vi "SyntaxCheck.vi"(8 "error in":errorcluster, 11 "Logical Parsed Expression":T1) -> (0 "error out":errorcluster, 1 "Error Index":i32, 2 "Funcion Analizada":string, 3 "Logical Parsed Expression Out":T1)   [LabVIEW 2014, in "SeqLoop.lvlib"]
uses:
  TypeDefs/LogicParsedExpression.ctl
  <vilib>/regexp/Match Regular Expression.xnode
  SeqLoop.lvlib
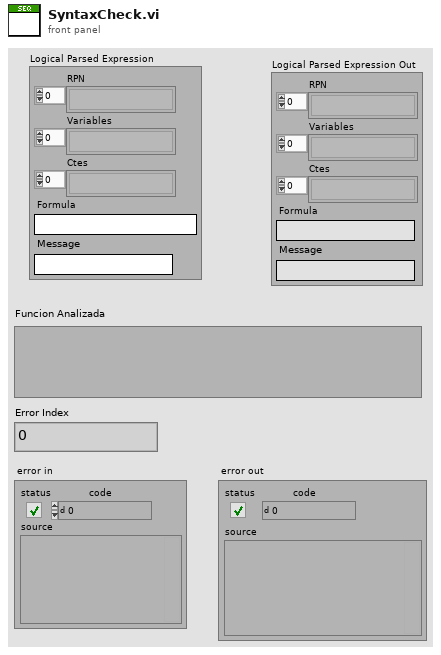
[diagram p1: front panel]
types:
  T1 = typedef "SeqLoop.lvlib/LogicParsedExpression.ctl" = cluster{"RPN ":string[], "Variables":string[], "Ctes":string[], "Formula":string, "Message":string}
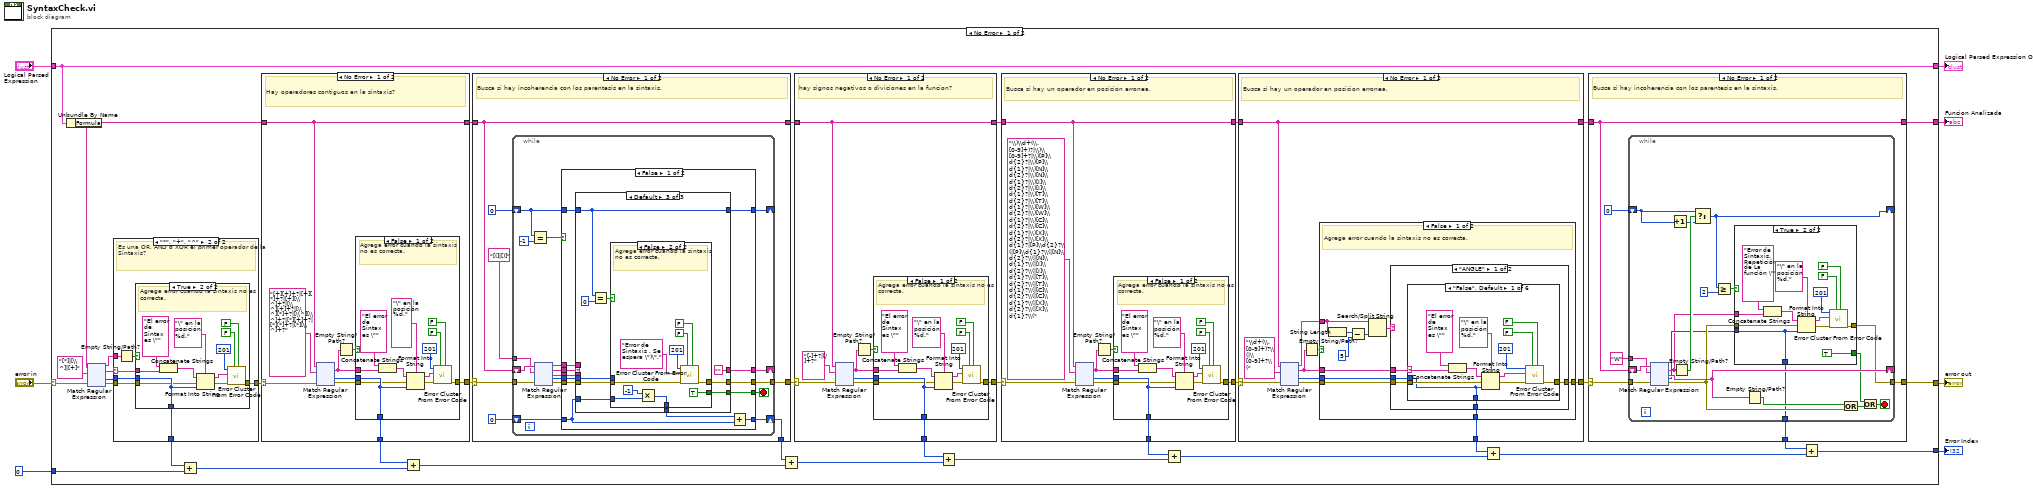
[diagram p0: block diagram]
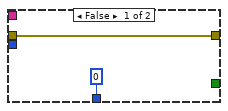
[diagram p2: hidden frame]
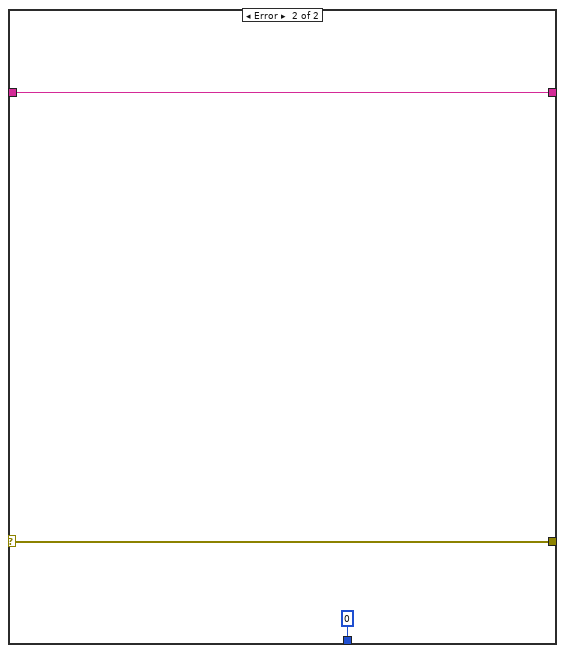
[diagram p3: hidden frame]
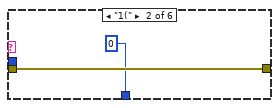
[diagram p4: hidden frame]
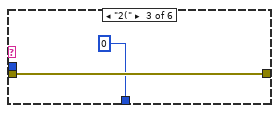
[diagram p5: hidden frame]
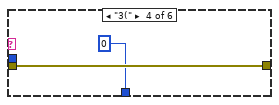
[diagram p6: hidden frame]
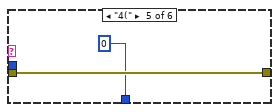
[diagram p7: hidden frame]
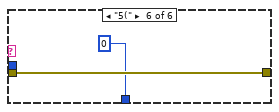
[diagram p8: hidden frame]
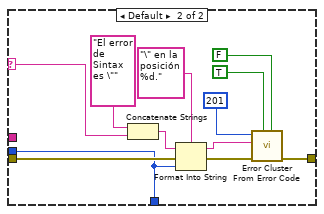
[diagram p9: hidden frame]
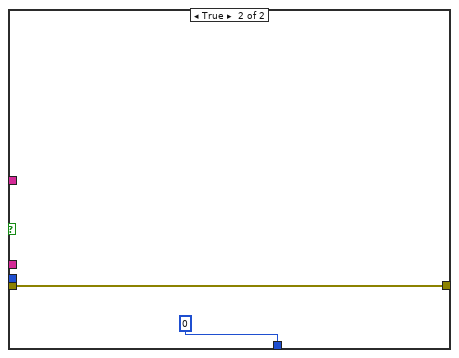
[diagram p10: hidden frame]
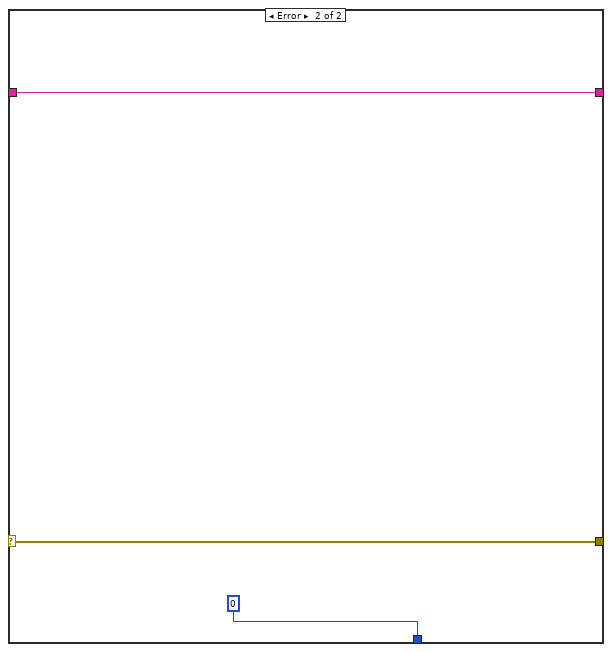
[diagram p11: hidden frame]
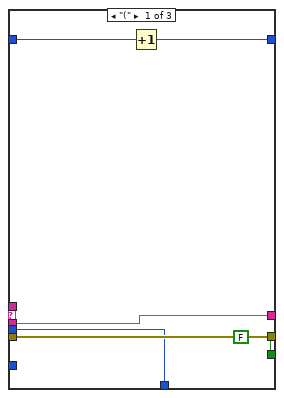
[diagram p12: hidden frame]
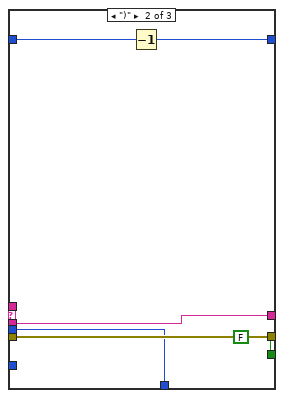
[diagram p13: hidden frame]
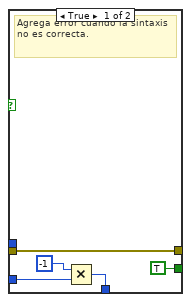
[diagram p14: hidden frame]
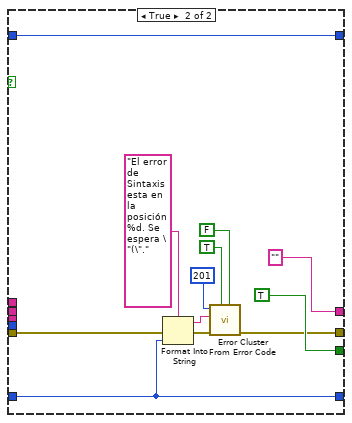
[diagram p15: hidden frame]
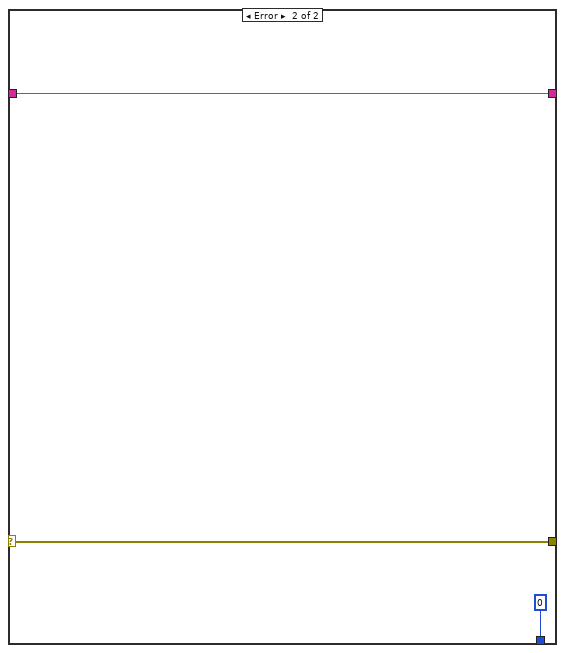
[diagram p16: hidden frame]
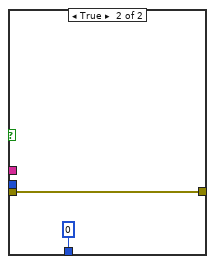
[diagram p17: hidden frame]
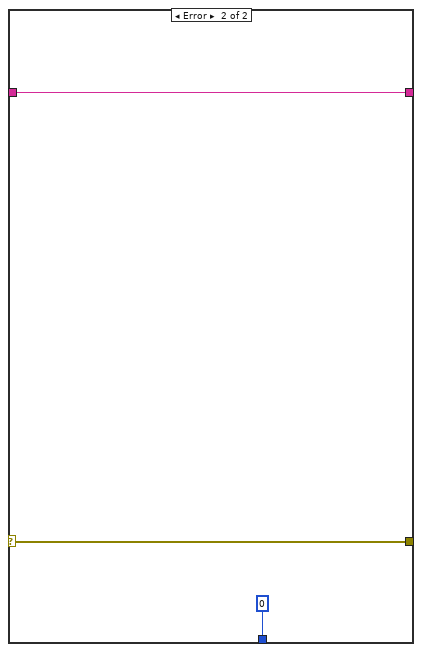
[diagram p18: hidden frame]
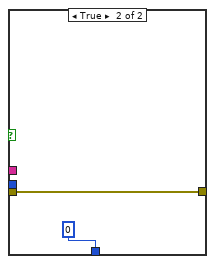
[diagram p19: hidden frame]
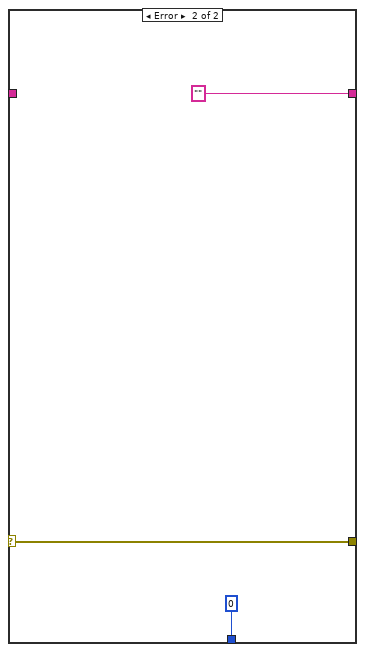
[diagram p20: hidden frame]
diagram:
  n1 = case shown="No Error" "error in" {
    selector: "error in" -> [w39 w1142]
    tunnel: [w12 w1142] -> w7
    tunnel: 0 ("Error Index") -> [w36 _]
    tunnel: "Logical Parsed Expression" -> [w31 w1141]
    tunnel: [w31 w1141] -> w1
    tunnel: [w11 ""] -> w4
    tunnel: [w8 0] -> w3
    frame No Error {
      n2 = Unbundle By Name(w31) -> ("Formula"=w32:string)
      n3 = xnode "Match Regular Expression"("input string"=w32, "regular expression"="[*]|[\\^]|[+]", "error in"=w39) -> ("before match"=w43:string, "whole match"=w42:string, "offset past match"=w37:i32, "error out"=w41:errorcluster)  [unwired: 3 in, 1 out]
      n4 = case shown="\"*\", \"+\", \"^\"" w42 {
        selector: w42 -> [_ w1008]
        tunnel: w41 -> [w1003 w1010]
        tunnel: [w1003 w1009] -> w38
        tunnel: w43 -> [_ w1006]
        tunnel: w37 -> [_ w1005]
        tunnel: [0 ("offset past match") w1004] -> w19
        frame Default {
        }
        frame "*", "+", "^" {
          # "Es una OR, AND o XOR el primer operador de la Sintaxis?"
          n5 = Empty String/Path?(string/path=w1006) -> (empty?=w1007:bool)
          n6 = case shown="True" w1007 {
            tunnel: w1010 -> [w1012 w1015]
            tunnel: [w1012 w1013] -> w1009
            tunnel: w1008 -> [_ w1014]
            tunnel: w1005 -> [_ w1016]
            tunnel: [0 ("offset past match") w1016] -> w1004
            frame False {
            }
            frame True {
              # "Agrega error cuando la sintaxis no es correcta."
              n7 = Concatenate Strings("El error de Sintax es \"" ("error message (\"\")"), w1014) -> (w1023:string)
              n8 = Format Into String(format string="\" en la posición %d.", initial string=w1023, error in=w1015, w1016) -> (resulting string=w1022:string, error out=w1021:errorcluster)
              n9 = call <vilib>:"Error Cluster From Error Code.vi"("is warning? (False)"=FALSE, "show call chain? (False)"=FALSE, "error in (no error)"=w1021, "error message (\"\")"=w1022, "error code (0)"=201) -> ("error out"=w1013:errorcluster)  [unwired: 4 in]
            }
          }
        }
      }
      n10 = Add(x=w19, y=w36) -> (x+y=w35:i32)
      n11 = case shown="No Error" w38 {
        selector: w38 -> [w866 w1001]
        tunnel: [w864 w1001] -> w25
        tunnel: w32 -> [w865 _]
        tunnel: [w865 "" ("String In")] -> w24
        tunnel: [w862 0 ("offset past match")] -> w34
        frame No Error {
          # "Hay operadores contiguos en la sintaxis?"
          n12 = xnode "Match Regular Expression"("input string"=w865, "regular expression"="[+][+]+?|[+][*]+?|[+][\\^]+?|[\\^][+]+?|[\\^][*]+?|[\\^][\\^]+?|[*][+]+?|[*][*]+?|[*][\\^]+?", "error in"=w866) -> ("whole match"=w868:string, "offset past match"=w863:i32, "error out"=w869:errorcluster)  [unwired: 3 in, 2 out]
          n13 = Empty String/Path?(string/path=w868) -> (empty?=w867:bool)
          n14 = case shown="False" w867 {
            tunnel: w869 -> [w875 w884]
            tunnel: [w881 w884] -> w864
            tunnel: w868 -> [w878 _]
            tunnel: w863 -> [w876 _]
            tunnel: [w876 0 ("offset past match")] -> w862
            frame False {
              # "Agrega error cuando la sintaxis no es correcta."
              n15 = Concatenate Strings("El error de Sintax es \"" ("error message (\"\")"), w878) -> (w872:string)
              n16 = Format Into String(format string="\" en la posición %d.", initial string=w872, error in=w875, w876) -> (resulting string=w873:string, error out=w874:errorcluster)
              n17 = call <vilib>:"Error Cluster From Error Code.vi"("is warning? (False)"=FALSE, "show call chain? (False)"=FALSE, "error in (no error)"=w874, "error message (\"\")"=w873, "error code (0)"=201) -> ("error out"=w881:errorcluster)  [unwired: 4 in]
            }
            frame True {
            }
          }
        }
        frame Error {
        }
      }
      n18 = Add(x=w34, y=w35) -> (x+y=w22:i32)
      n19 = case shown="No Error" w25 {
        selector: w25 -> [w384 w581]
        tunnel: [w385 w581] -> w26
        tunnel: w24 -> [w380 w580]
        tunnel: [w380 w580] -> w23
        tunnel: [w379 0] -> w20
        frame No Error {
          # "Busca si hay incoherencia con los parentesis en la sintaxis."
          n20 = while {
            tunnel: "[(]|[)]" ("regular expression") -> [w399]
            shift-right: [w400] -> _
            shift-left: w380 -> [w402]
            tunnel: w384 -> [w401]
            tunnel: [w394] -> w385
            shift-right: [w395] -> _
            shift-left: 0 -> [w389]
            shift-right: [w386] -> w379
            shift-left: 0 -> [w387]
            stop <- w393 stop-if-true
            n21 = Equal?(x=w389, y=-1) -> (x = y?=w390:bool)
            n22 = xnode "Match Regular Expression"("input string"=w402, "regular expression"=w399, "error in"=w401) -> ("before match"=w396:string, "whole match"=w391:string, "after match"=w398:string, "offset past match"=w392:i32, "error out"=w397:errorcluster)  [unwired: 3 in]
            n23 = case shown="False" w390 {
              tunnel: [w415 "" ("after match")] -> w400
              tunnel: w398 -> [w414 _]
              tunnel: w397 -> [w413 w462]
              tunnel: w396 -> [w412 _]
              tunnel: w389 -> [w411 w455]
              tunnel: [w410 w455] -> w395
              tunnel: [w409 w463] -> w394
              tunnel: [w408 TRUE] -> w393
              tunnel: w392 -> [w407 _]
              tunnel: w391 -> [w406 _]
              tunnel: w387 -> [w403 w453]
              tunnel: [w404 w453] -> w386
              frame False {
                n24 = case shown="Default" w406 {
                  tunnel: [w421 w427 "" ("after match")] -> w415
                  tunnel: w412 -> [_ _ _]
                  tunnel: w414 -> [w421 w427 _]
                  tunnel: w413 -> [w420 w426 w437]
                  tunnel: [w420 w426 w436] -> w409
                  tunnel: [FALSE FALSE w434] -> w408
                  tunnel: w411 -> [w419 w425 w432]
                  tunnel: [w418 w424 w432] -> w410
                  tunnel: w407 -> [w416 w422 w433]
                  tunnel: [w416 w422 w431] -> w405
                  tunnel: w403 -> [_ _ w428]
                  frame "(" {
                    n25 = Increment(x=w419) -> (x+1=w418:i32)
                  }
                  frame ")" {
                    n26 = Decrement(x=w425) -> (x-1=w424:i32)
                  }
                  frame Default {
                    n27 = Equal?(x=w432, y=0) -> (x = y?=w430:bool)
                    n28 = case shown="False" w430 {
                      tunnel: w437 -> [w441 w446]
                      tunnel: [w441 w448] -> w436
                      tunnel: [TRUE TRUE] -> w434
                      tunnel: w433 -> [_ _]
                      tunnel: [w439 w444] -> w431
                      tunnel: w428 -> [w438 w445]
                      frame True {
                        # "Agrega error cuando la sintaxis no es correcta."
                        n29 = Multiply(x=-1 ("offset past match"), y=w438) -> (x*y=w439:i32)
                      }
                      frame False {
                        # "Agrega error cuando la sintaxis no es correcta."
                        n30 = Multiply(x=-1, y=w445) -> (x*y=w444:i32)
                        n31 = call <vilib>:"Error Cluster From Error Code.vi"("is warning? (False)"=FALSE, "show call chain? (False)"=FALSE, "error in (no error)"=w446, "error message (\"\")"="Error de Sintaxis . Se espera \")\"." ("format string"), "error code (0)"=201) -> ("error out"=w448:errorcluster)  [unwired: 4 in]
                      }
                    }
                  }
                }
                n32 = Add(x=w405, y=w403) -> (x+y=w404:i32)
              }
              frame True {
                n33 = Format Into String(format string="El error de Sintaxis  esta en la posición %d. Se espera \"(\".", error in=w462, w453) -> (resulting string=w457:string, error out=w458:errorcluster)  [unwired: 1 in]
                n34 = call <vilib>:"Error Cluster From Error Code.vi"("is warning? (False)"=FALSE, "show call chain? (False)"=TRUE, "error in (no error)"=w458, "error message (\"\")"=w457, "error code (0)"=201) -> ("error out"=w463:errorcluster)  [unwired: 4 in]
              }
            }
          }
        }
        frame Error {
        }
      }
      n35 = Add(x=w20, y=w22) -> (x+y=w21:i32)
      n36 = case shown="No Error" w26 {
        selector: w26 -> [w730 w861]
        tunnel: [w727 w861] -> w30
        tunnel: w23 -> [w729 _]
        tunnel: [w729 "" ("String In")] -> w29
        tunnel: [w722 0 ("offset past match")] -> w33
        frame No Error {
          # "hay signos negativos o diviciones en la funcion?"
          n37 = xnode "Match Regular Expression"("input string"=w729, "regular expression"="[-]+?|[/]+?", "error in"=w730) -> ("whole match"=w725:string, "offset past match"=w723:i32, "error out"=w724:errorcluster)  [unwired: 3 in, 2 out]
          n38 = Empty String/Path?(string/path=w725) -> (empty?=w726:bool)
          n39 = case shown="False" w726 {
            tunnel: w724 -> [w735 w744]
            tunnel: [w741 w744] -> w727
            tunnel: w725 -> [w738 _]
            tunnel: w723 -> [w736 _]
            tunnel: [w736 0 ("offset past match")] -> w722
            frame False {
              # "Agrega error cuando la sintaxis no es correcta."
              n40 = Concatenate Strings("El error de Sintax es \"" ("error message (\"\")"), w738) -> (w732:string)
              n41 = Format Into String(format string="\" en la posición %d.", initial string=w732, error in=w735, w736) -> (resulting string=w733:string, error out=w734:errorcluster)
              n42 = call <vilib>:"Error Cluster From Error Code.vi"("is warning? (False)"=FALSE, "show call chain? (False)"=FALSE, "error in (no error)"=w734, "error message (\"\")"=w733, "error code (0)"=201) -> ("error out"=w741:errorcluster)  [unwired: 4 in]
            }
            frame True {
            }
          }
        }
        frame Error {
        }
      }
      n43 = Add(x=w33, y=w21) -> (x+y=w27:i32)
      n44 = case shown="No Error" w30 {
        selector: w30 -> [w585 w721]
        tunnel: w29 -> [w584 w720]
        tunnel: [w586 w721] -> w18
        tunnel: [w584 w720] -> w17
        tunnel: [w582 0 ("offset past match")] -> w28
        frame No Error {
          # "Busca si hay un operador en posicion erronea."
          n45 = xnode "Match Regular Expression"("input string"=w584, "regular expression"="\\)\\d+(\\.[0-9]+)?|\\)\\[0-9]+?|\\)[P]\\d{2}?|\\)[P]\\d{1}?|\\)[N]\\d{2}?|\\)[N]\\d{1}?|\\)[I]\\d{2}?|\\)[I]\\d{1}?|\\)[T]\\d{2}?|\\)[T]\\d{1}?|\\)[W]\\d{2}?|\\)[W]\\d{1}?|\\)[C]\\d{2}?|\\)[C]\\d{1}?|\\)[X]\\d{2}?|\\)[X]\\d{1}?|[P]\\d{2}?\\(|[P]\\d{1}?\\(|[N]\\d{2}?\\(|[N]\\d{1}?\\(|[I]\\d{2}?\\(|[I]\\d{1}?\\(|[T]\\d{2}?\\(|[T]\\d{1}?\\(|[C]\\d{2}?\\(|[C]\\d{1}?\\(|[X]\\d{2}?\\(|[X]\\d{1}?\\(", "error in"=w585) -> ("whole match"=w588:string, "offset past match"=w590:i32, "error out"=w589:errorcluster)  [unwired: 3 in, 2 out]
          n46 = Empty String/Path?(string/path=w588) -> (empty?=w587:bool)
          n47 = case shown="False" w587 {
            tunnel: w589 -> [w595 w604]
            tunnel: [w601 w604] -> w586
            tunnel: w588 -> [w598 _]
            tunnel: w590 -> [w596 _]
            tunnel: [w596 0 ("offset past match")] -> w582
            frame False {
              # "Agrega error cuando la sintaxis no es correcta."
              n48 = Concatenate Strings("El error de Sintax es \"" ("error message (\"\")"), w598) -> (w592:string)
              n49 = Format Into String(format string="\" en la posición %d.", initial string=w592, error in=w595, w596) -> (resulting string=w593:string, error out=w594:errorcluster)
              n50 = call <vilib>:"Error Cluster From Error Code.vi"("is warning? (False)"=FALSE, "show call chain? (False)"=FALSE, "error in (no error)"=w594, "error message (\"\")"=w593, "error code (0)"=201) -> ("error out"=w601:errorcluster)  [unwired: 4 in]
            }
            frame True {
            }
          }
        }
        frame Error {
        }
      }
      n51 = Add(x=w28, y=w27) -> (x+y=w16:i32)
      n52 = case shown="No Error" w18 {
        selector: w18 -> [w204 w378]
        tunnel: w17 -> [w202 w377]
        tunnel: [w203 w378] -> w13
        tunnel: [w202 w377] -> w14
        tunnel: [w201 0 ("offset past match")] -> w15
        frame No Error {
          # "Busca si hay un operador en posicion erronea."
          n53 = xnode "Match Regular Expression"("input string"=w202, "regular expression"="\\d+(\\.[0-9]+)?\\(|\\[0-9]+?\\(", "error in"=w204) -> ("before match"=w205:string, "whole match"=w208:string, "offset past match"=w210:i32, "error out"=w209:errorcluster)  [unwired: 3 in, 1 out]
          n54 = Empty String/Path?(string/path=w208) -> (empty?=w207:bool)
          n55 = case shown="False" w207 {
            tunnel: w209 -> [w218 w261]
            tunnel: [w220 w261] -> w203
            tunnel: w208 -> [w219 _]
            tunnel: w210 -> [w217 _]
            tunnel: [w216 0 ("offset past match")] -> w201
            tunnel: w205 -> [w212 _]
            frame False {
              # "Agrega error cuando la sintaxis no es correcta."
              n56 = String Length(string=w212) -> (length=w213:i32)
              n57 = Subtract(x=w213, y=5) -> (x-y=w215:i32)
              n58 = Search/Split String(string=w212, offset (0)=w215) -> (match + rest of string=w211:string)  [unwired: 1 in, 2 out]
              n59 = case shown="\"ANGLE\"" w211 {
                selector: w211 -> [_ w248]
                tunnel: [w224 w258] -> w220
                tunnel: w219 -> [w223 _]
                tunnel: w217 -> [w221 w250]
                tunnel: w218 -> [w225 w255]
                tunnel: [w222 w250] -> w216
                frame "ANGLE" {
                  n60 = case shown="\"False\", Default" w223 {
                    selector: w223 -> [w227 _ _ _ _ _]
                    tunnel: w225 -> [w228 w239 w241 w243 w245 w247]
                    tunnel: [w229 w239 w241 w243 w245 w247] -> w224
                    tunnel: [w226 0 ("offset past match") 0 ("offset past match") 0 ("offset past match") 0 ("offset past match") 0 ("offset past match")] -> w222
                    tunnel: w221 -> [w226 _ _ _ _ _]
                    frame "False", Default {
                      n61 = Concatenate Strings("El error de Sintax es \"" ("error message (\"\")"), w227) -> (w232:string)
                      n62 = Format Into String(format string="\" en la posición %d.", initial string=w232, error in=w228, w226) -> (resulting string=w233:string, error out=w234:errorcluster)
                      n63 = call <vilib>:"Error Cluster From Error Code.vi"("is warning? (False)"=FALSE, "show call chain? (False)"=FALSE, "error in (no error)"=w234, "error message (\"\")"=w233, "error code (0)"=201) -> ("error out"=w229:errorcluster)  [unwired: 4 in]
                    }
                    frame "1(" {
                    }
                    frame "2(" {
                    }
                    frame "3(" {
                    }
                    frame "4(" {
                    }
                    frame "5(" {
                    }
                  }
                }
                frame Default {
                  n64 = Concatenate Strings("El error de Sintax es \"" ("error message (\"\")"), w248) -> (w252:string)
                  n65 = Format Into String(format string="\" en la posición %d.", initial string=w252, error in=w255, w250) -> (resulting string=w253:string, error out=w254:errorcluster)
                  n66 = call <vilib>:"Error Cluster From Error Code.vi"("is warning? (False)"=FALSE, "show call chain? (False)"=TRUE, "error in (no error)"=w254, "error message (\"\")"=w253, "error code (0)"=201) -> ("error out"=w258:errorcluster)  [unwired: 4 in]
                }
              }
            }
            frame True {
            }
          }
        }
        frame Error {
        }
      }
      n67 = Add(x=w15, y=w16) -> (x+y=w9:i32)
      n68 = case shown="No Error" w13 {
        selector: w13 -> [w48 w200]
        tunnel: [w49 w200] -> w12
        tunnel: w14 -> [w45 w199]
        tunnel: [w45 w199] -> w11
        tunnel: [w44 0 ("offset past match")] -> w10
        frame No Error {
          # "Busca si hay incoherencia con los parentesis en la sintaxis."
          n69 = while {
            tunnel: "W" ("regular expression") -> [w66]
            shift-right: [w63] -> _
            shift-left: w45 -> [w68]
            tunnel: w48 -> [w67]
            tunnel: [w53] -> w49
            shift-right: [w59] -> _
            shift-left: 0 -> [w61]
            tunnel: [w50] -> w44
            stop <- w56 stop-if-true
            n70 = xnode "Match Regular Expression"("input string"=w68, "regular expression"=w66, "error in"=w67) -> ("whole match"=w51:string, "after match"=w63:string, "offset past match"=w52:i32, "error out"=w54:errorcluster)  [unwired: 3 in, 1 out]
            n71 = Increment(x=w61) -> (x+1=w62:i32)
            n72 = Empty String/Path?(string/path=w51) -> (empty?=w65:bool)
            n73 = Select(t=w61, s=w65, f=w62) -> (s? t:f=w59:i32)
            n74 = Greater Or Equal?(x=w59, y=2) -> (x >= y?=w58:bool)
            n75 = case shown="True" w58 {
              tunnel: [_ TRUE ("x .or. y?")] -> w55
              tunnel: w54 -> [w70 w74]
              tunnel: [w70 w73] -> w53
              tunnel: w52 -> [_ w71]
              tunnel: w51 -> [_ w72]
              tunnel: [0 ("offset past match") w71] -> w50
              frame False {
              }
              frame True {
                n76 = Concatenate Strings("Error de Sintaxis. Repetición de La función \"" ("error message (\"\")"), w72) -> (w80:string)
                n77 = Format Into String(format string="\" en la posición %d.", initial string=w80, error in=w74, w71) -> (resulting string=w79:string, error out=w78:errorcluster)
                n78 = call <vilib>:"Error Cluster From Error Code.vi"("is warning? (False)"=FALSE, "show call chain? (False)"=FALSE, "error in (no error)"=w78, "error message (\"\")"=w79, "error code (0)"=201) -> ("error out"=w73:errorcluster)  [unwired: 4 in]
              }
            }
            n79 = Empty String/Path?(string/path=w63) -> (empty?=w64:bool)
            n80 = Or(x=w64, y=w54) -> (x .or. y?=w57:bool)
            n81 = Or(x=w55, y=w57) -> (x .or. y?=w56:bool)
          }
        }
        frame Error {
        }
      }
      n82 = Add(x=w10, y=w9) -> (x+y=w8:i32)
    }
    frame Error {
    }
  }
  "error out" <- w7
  "Funcion Analizada" <- w4
  "Error Index" <- w3
  "Logical Parsed Expression Out" <- w1
